vi "StellarNet_Raman_Obtain_Spectra_MODIFIED.vi"() -> ()   [LabVIEW 2014]
uses:
  Environmental Chamber LabVIEW and Instruments/Environment_Instrument_VIs/SpectraWiz_LabVIEW-1chan-free 2013.llb/StellarNet SpectraWiz Globals.vi
panel:
  in  "Channel to monitor":i8=1 min=1 max=1
  out "?":T1(graph)
  in  "Use Dark":bool
  in  "Take Dark":bool
  in  "Take Reference":bool
  in  "Mode Selection":u16(ring) items=["Scope Mode", "Absorbance Mode", "Transmission Mode", "Radiometer Mode"]
  in  "View Data File":bool
  in  "Open Data File":bool
  out "?":T1(graph)
  in  "Reset Coefficients":bool
  in  "Drift Correct":bool
  in  "View Snapshot":bool
  in  "Take Snapshot":bool
  in  "Channel":u8=1 min=1 max=1
  in  "Operating Parameters":T2(array[cluster]) {"Digitizer Clock Rate Setting" min=1 max=3; "Optical Smoothing Level" min=0 max=4 step=1; "Number of Scans to Average" min=1 max=10000 step=1}
  out "Number of Channels:":i32
  in  "Clear History":bool
  out "?":T1(graph)
  in  "Create and Log to Time Series Log File":bool
  out "ChartView":T3(graph)
  out "Time [s]":dbl format="%.2f"
  out "Data File":cluster{dbl[], dbl[]}
  out "Cursor Indices":i32[](array[numeric])
  in  "Stop Program":bool
  # "``"
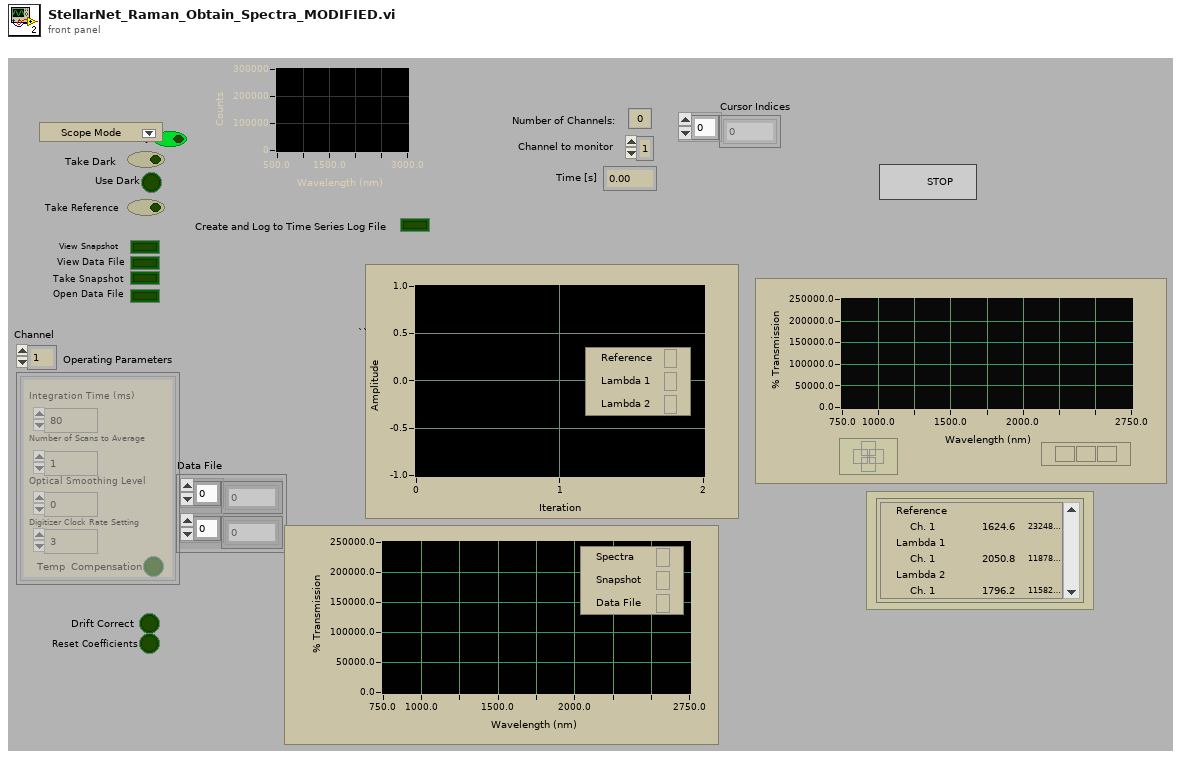
[diagram p1: front panel]
types:
  T1 = cluster{"Spectrometer Wavelengths":dbl[], dbl[]}[]
  T2 = cluster{"Integration Time (ms)":i32, "Number of Scans to Average":i32, "Optical Smoothing Level":i32, "Digitizer Clock Rate Setting":i32, "Temp  Compensation ":bool}[]
  T3 = cluster{"Cursor Y":dbl, "Cursor Y":dbl, "Cursor Y":dbl}
  T4 = cluster{"Cursor Y":dbl, "Cursor Y":dbl, "Cursor Y":dbl}[]
  T5 = cluster{"Coefficients":ext[], "Wavelengths":dbl[]}[]
  T6 = cluster{"[0]":dbl, "[1]":dbl, "[2]":dbl, "[3]":dbl, "[4]":dbl, "[5]":dbl, "[6]":dbl, "[7]":dbl, "[8]":dbl}
  T7 = cluster{"Minimum":dbl, "Maximum":dbl, "Increment":dbl, "Minor Incr":dbl, "Start":dbl}
  T8 = cluster{"Integration Time (ms)":i32, "Number of Scans to Average":i32, "Optical Smoothing Level":i32, "Digitizer Clock Rate Setting":i32, "Temp  Compensation ":bool}
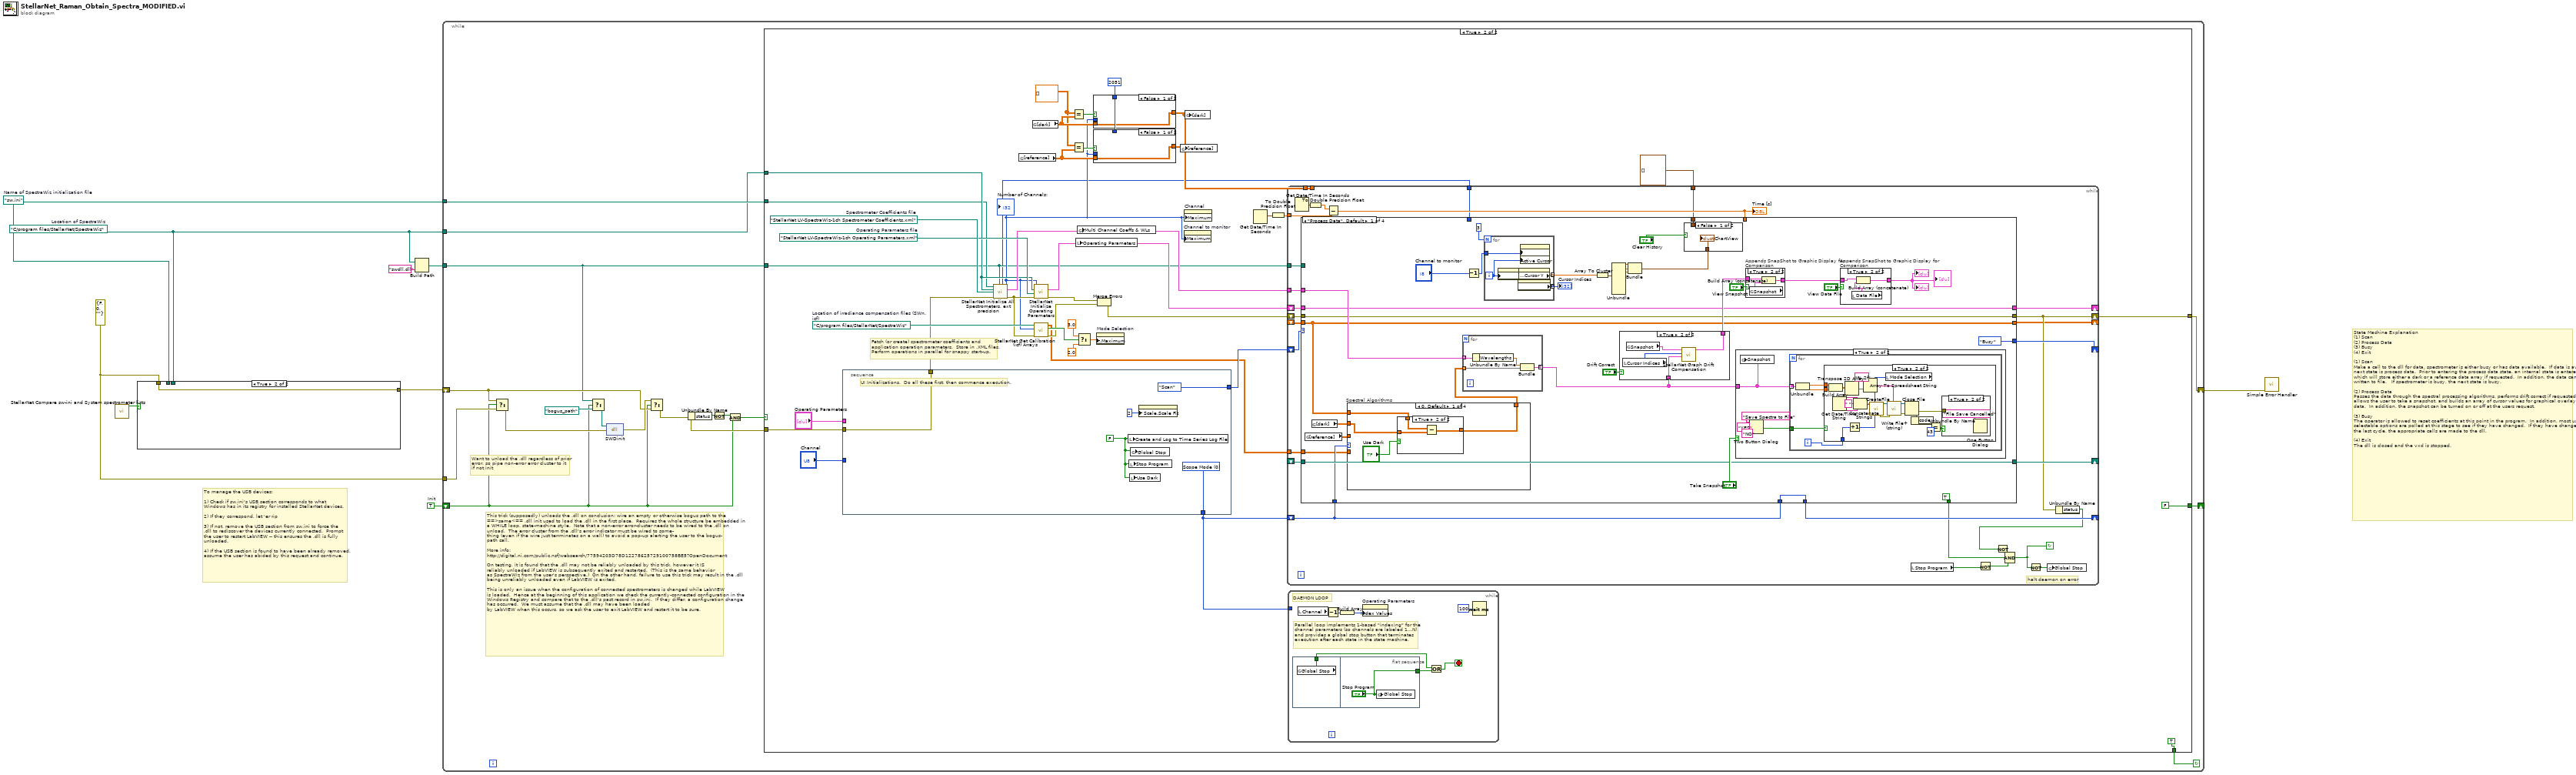
[diagram p0: block diagram]
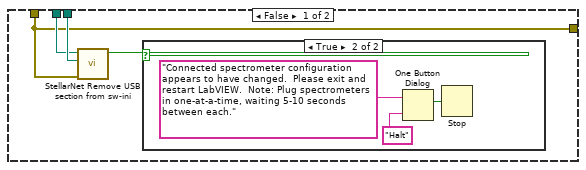
[diagram p2: hidden frame]
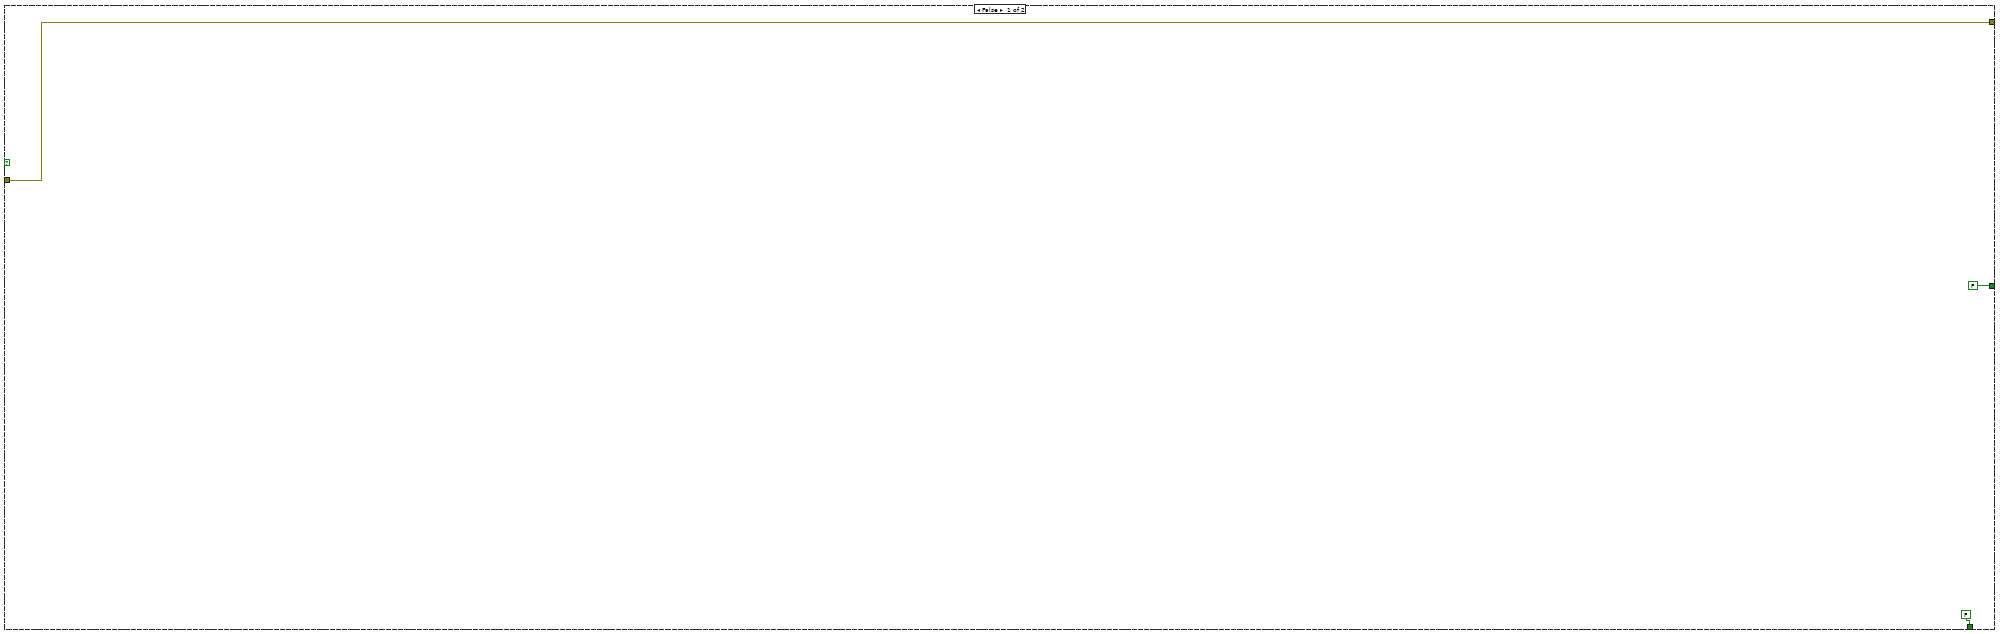
[diagram p4: hidden frame]
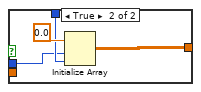
[diagram p5: hidden frame]
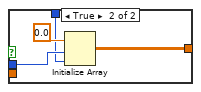
[diagram p6: hidden frame]
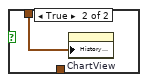
[diagram p7: hidden frame]
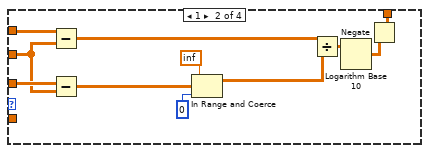
[diagram p12: hidden frame]
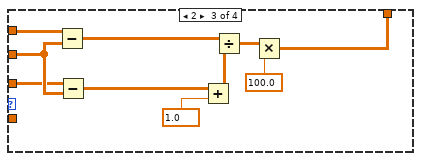
[diagram p13: hidden frame]
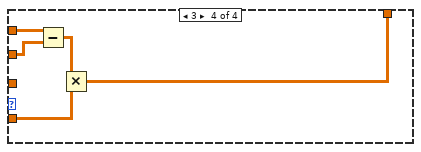
[diagram p14: hidden frame]
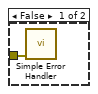
[diagram p17: hidden frame]
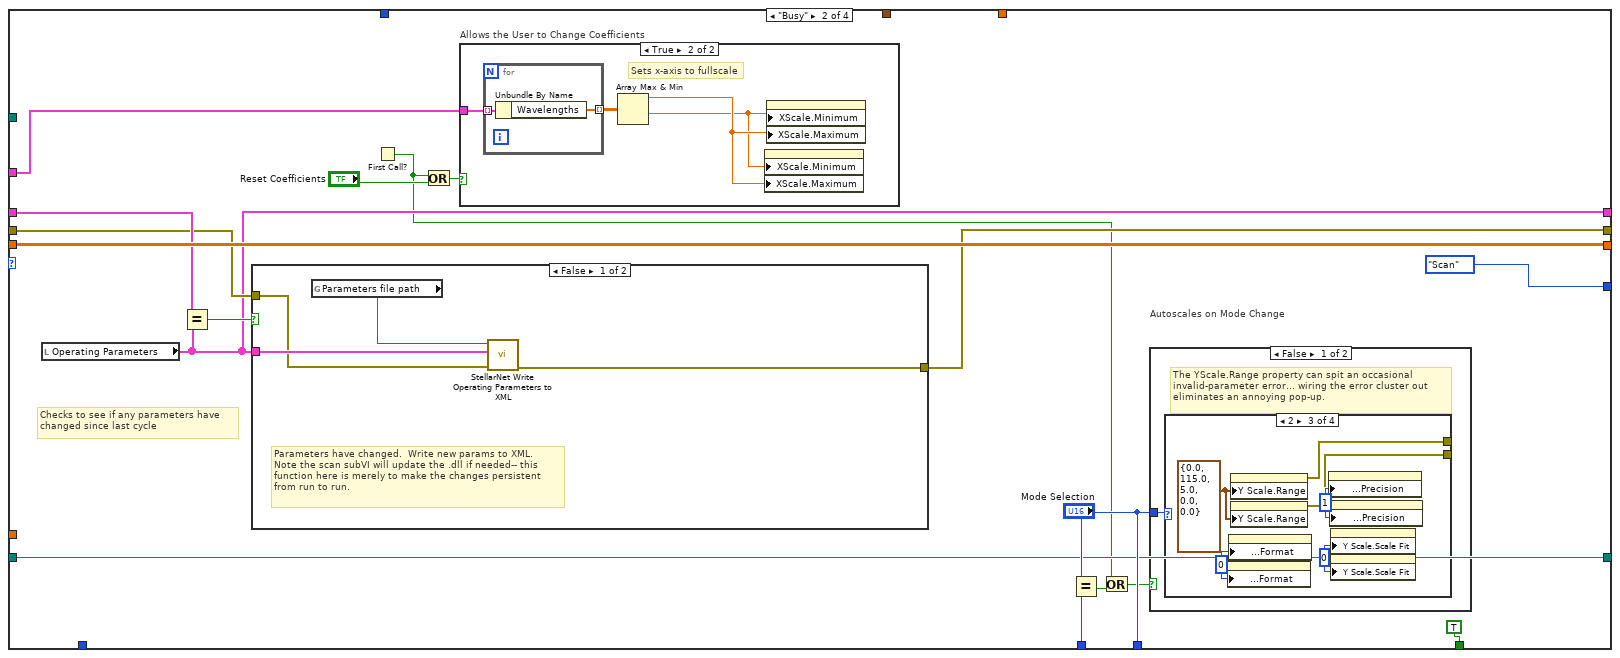
[diagram p18: hidden frame]
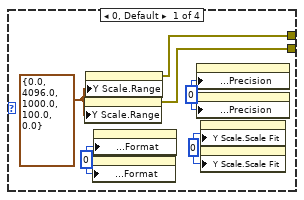
[diagram p20: hidden frame]
diagram:
  w4 = path "C:/program files/StellarNet/SpectraWiz"  # Location of SpectraWiz
  w8 = path "sw.ini"  # Name of SpectraWiz initialization file
  w6 = errorcluster {"status"=FALSE, "code"=0, "source"=""} ("error in (no error)")
  w9 = TRUE  # Init
  # "To manage the USB devices:\n\n1) Check if sw.ini's USB section corresponds to what\nWindows has in its registry for installed StellarNet devices.\n\n2) If they correspond, let 'er rip\n\n3) If not, remove the USB section from sw.ini to force the \n.dll to rediscover the devices currently connected.  Prompt\nthe user to restart LabVIEW -- this ensures the .dll is fully\nunloaded.  \n\n4) If the USB section is found to have been already removed, \nassume the user has abided by this request and continue."
  # "State Machine Explanation\n(1) Scan\n(2) Process Data\n(3) Busy\n(4) Exit\n\n(1) Scan\nMake a call to the dll for data, spectrometer is either busy or has data available.  If data is available, next state is process data.  Prior to entering the process data state, an internal state is entered which will store either a dark or a reference data array if requested.  In addition, the data can be written to file.   If spectrometer is busy, the next state is busy.\n\n(2) Process Data\nPasses the data through the spectral processing algorithms, performs drift correct if requested, allows the user to take a snapshot, and builds an array of cursor values for graphical overlay on the data.  In addition, the snapshot can be turned on or off at the users request.\n\n(3) Busy\nThe operator is allowed to reset coefficients at this point in the program.  In addition, most user selectable options are polled at this stage to see if they have changed.  If they have changed since the last cycle, the appropriate calls are made to the dll.\n\n(4) Exit\nThe dll is closed and the vxd is stopped."
  n1 = call "StellarNet Compare sw-ini and System spectrometer lists.vi"() -> ("Configs\nAgree"=w5:bool)  [unwired: 11 in]
  n2 = case shown="True" w5 {
    tunnel: w6 -> [w11 w17]
    tunnel: w4 -> [w13 _]
    tunnel: w8 -> [w12 _]
    tunnel: [w11 w17] -> w7
    frame False {
      n3 = call "StellarNet Remove USB section from sw-ini.vi"("error in (no error)"=w11, "Location of SpectraWiz"=w13, "Name of SpectraWiz initialization file"=w12) -> ("USB section found?"=w10:bool)  [unwired: 7 in, 1 out]
      n4 = case shown="True" w10 {
        frame False {
        }
        frame True {
          n5 = One Button Dialog(message="Connected spectrometer configuration appears to have changed.  Please exit and restart LabVIEW.  Note: Plug spectrometers in one-at-a-time, waiting 5-10 seconds between each.", button name ("OK")="Halt") -> (true=w15:bool)
          n6 = Stop(stop? (T)=w15) -> ()
        }
      }
    }
    frame True {
    }
  }
  n7 = Build Path(base path=w4, name or relative path="swdll.dll") -> (appended path=w2:path)
  n8 = while {
    shift-right: [w34] -> _
    shift-left: w9 -> [w20]
    tunnel: w8 -> [w27]
    tunnel: w4 -> [w19]
    shift-right: [w26] -> w1
    shift-left: w7 -> [w21]
    tunnel: w6 -> [w25]
    tunnel: w2 -> [w18]
    stop <- w33 continue-if-true
    # "This trick (supposedly) unloads the .dll on conclusion: wire an empty or otherwise bogus path to the ==>same<== .dll init used to load the .dll in the first place.  Requires the whole structure be embedded in a WHILE loop, state-machine style.  Note that a non-error error-cluster needs to be wired to the .dll on unload.  The error cluster from the .dll's error indicator must be wired to some-\nthing (even if the wire just terrminates on a wall) to avoid a pop-up alerting the user to the bogus-\npath call.\n\nMore info:\nhttp://digital.ni.com/public.nsf/websearch/77594203D78D12278625729100758BE5?OpenDocument\n\nOn testing, it is found that the .dll may not be reliably unloaded by this trick, however it IS\nreliably unloaded if LabVIEW is subsequently exited and restarted.  (This is the same behavior\nas SpectraWiz from the user's perspective.)  On the other hand, failure to use this trick may result in the .dll being unreliably unloaded even if LabVIEW is exited.\n\nThis is only an issue when the configuration of connected spectrometers is changed while LabVIEW\nis loaded.  Hence at the beginning of this application we check the currently-connected configuration in the Windows Registry and compare that to the .dll's past record in sw.ini.  If they differ, a configuration change has occurred.  We must assume that the .dll may have been loaded \nby LabVIEW when this occurs, so we ask the user to exit LabVIEW and restart it to be sure."
    # "Want to unload the .dll regardless of prior\nerror, so pipe non-error error cluster to it\nif not init"
    n9 = Select(t=w21, s=w20, f=w25) -> (s? t:f=w24:errorcluster)
    n10 = Select(t=w18, s=w20, f=path "bogus_path" ("reference")) -> (s? t:f=w31:path)
    n11 = dll-call lib="C:/Program Files/StellarNet/SpectraWiz/swdll.dll" fn="SWDinit" label="init"(path in=w31, error in=w24) -> (error out=w23:errorcluster)  [unwired: 2 in, 1 out]
    n12 = Select(t=w23, s=w20, f=w21) -> (s? t:f=w22:errorcluster)
    n13 = Unbundle By Name(w22) -> ("status"=w29:bool)
    n14 = Not(x=w29) -> (.not. x?=w30:bool)
    n15 = And(x=w30, y=w20) -> (x .and. y?=w28:bool)
    n16 = case shown="True" w28 {
      tunnel: [w35 w42] -> w26
      tunnel: w22 -> [w35 w48]
      tunnel: [FALSE ("Init") FALSE ("Init")] -> w34
      tunnel: [FALSE TRUE] -> w33
      tunnel: w19 -> [_ w44]
      tunnel: w27 -> [_ w43]
      tunnel: w18 -> [_ w39]
      frame False {
      }
      frame True {
        w49 = 2051 ("dimension size")
        w54 = sgl[][] [] ("[dark]")
        w72 = path "C:/program files/StellarNet/SpectraWiz"  # Location of irradiance compensation files (SWn.icf)
        w73 = path "StellarNet LV-SpectraWiz-1ch Operating Parameters.xml"  # Operating Parameters file
        w74 = path "StellarNet LV-SpectraWiz-1ch Spectrometer Coefficients.xml"  # Spectrometer Coefficients file
        # "Fetch (or create) spectrometer coefficients and\napplication operation parameters.  Store in .XML files.\nPerform operations in parallel for snappy start-up."
        n17 = stacked-sequence {
          tunnel: [w99] -> w57
          tunnel: [enum16{"Process Data", "Busy", "Exit", "Scan"}."Scan" ("Enum")] -> w64
          tunnel: [w97] -> w45
          tunnel: "Channel" -> [_]
          tunnel: "Operating Parameters" -> [_]
          tunnel: w48 -> [w97]
          frame #0 {
            w99 = u16 0 items=["Scope Mode", "Absorbance Mode", "Transmission Mode", "Radiometer Mode"] ("Mode Selection")
            w96 = FALSE ("File Stamp")
            # "UI Initializations.  Do all these first, then commence execution."
            n18 = local write "Create and Log to Time Series Log File"(w96) -> ()
            n19 = local write "Stop Program"(w96) -> ()
            n20 = local write "Use Dark"(w96) -> ()
            n21 = global write "StellarNet SpectraWiz Globals.vi" "Global Stop"(w96) -> ()
            n22 = property class="XYGraph (strict)"("Y Scale.Scale Fit"=u8 2) -> ()  [unwired: 2 in, 2 out]
          }
        }
        n23 = call "StellarNet Initialize All Spectrometers, ext precision.vi"("Path of swdll.dll"=w39, "error in"=w45, "Spectrometer Coefficients file"=w74, "Location of SpectraWiz"=w44, "Name of SpectraWiz initialization file"=w43) -> ("error out"=w71:errorcluster, "Multi Channel Coeffs & WLs"=w58:T5, "Number of Channels"=w40:i32, "Detector Types"=w38:u16[])  [unwired: 2 in, 1 out]
        "Number of Channels:" <- w40
        n24 = global read "StellarNet SpectraWiz Globals.vi" "[reference]"() -> (w52:sgl[][])
        n25 = global read "StellarNet SpectraWiz Globals.vi" "[dark]"() -> (w55:sgl[][])
        n26 = call "StellarNet Initialize Operating Parameters.vi"("error in"=w71, "Spectrometer Coefficients file"=w73, "Location of SpectraWiz"=w44, "Number of Channels"=w40) -> ("error out"=w66:errorcluster, "Operating Parameters"=w61:T2)  [unwired: 6 in]
        n27 = call "StellarNet Get Calibration (icf) Arrays.vi"("error in (no error)"=w71, "Number of Channels"=w40, "directory path"=w72) -> ("error out"=w65:errorcluster, ".icf found for\nat least one channel"=w67:bool, "N x Compensation Array"=w62:dbl[][])  [unwired: 6 in]
        n28 = Equal?(x=w54, y=w55) -> (x = y?=w56:bool)
        n29 = Equal?(x=w54, y=w52) -> (x = y?=w53:bool)
        n30 = local write "Operating Parameters"(w61) -> ()
        n31 = global write "StellarNet SpectraWiz Globals.vi" "Multi Channel Coeffs & WLs"(w58) -> ()
        n32 = Select(t=3.0 ("Data Range:Maximum"), s=w67, f=2.0 ("Data Range:Maximum")) -> (s? t:f=w70:dbl)
        n33 = case shown="False" w56 {
          tunnel: [w82 w86] -> w51
          tunnel: w55 -> [w82 _]
          tunnel: w40 -> [_ w84]
          tunnel: w49 -> [_ w83]
          frame False {
          }
          frame True {
            n34 = Initialize Array(0.0, w84, w83) -> (w86:dbl[][])
          }
        }
        n35 = case shown="False" w53 {
          tunnel: [w77 w81] -> w50
          tunnel: w52 -> [w77 _]
          tunnel: w40 -> [_ w78]
          tunnel: w49 -> [_ w79]
          frame False {
          }
          frame True {
            n36 = Initialize Array(0.0, w78, w79) -> (w81:dbl[][])
          }
        }
        n37 = property on="Mode Selection" class="Ring (strict)"("Data Range:Maximum"=w70) -> ()  [unwired: 2 in, 2 out]
        n38 = Merge Errors(w66, w65) -> (w63:errorcluster)
        n39 = global write "StellarNet SpectraWiz Globals.vi" "[reference]"(w50) -> ()
        n40 = property on="Channel to monitor" class="DigNum (strict)"("Maximum"=w40) -> ()  [unwired: 2 in, 2 out]
        n41 = property on="Channel" class="DigNum (strict)"("Maximum"=w40) -> ()  [unwired: 2 in, 2 out]
        n42 = global write "StellarNet SpectraWiz Globals.vi" "[dark]"(w51) -> ()
        n43 = Get Date/Time In Seconds() -> (seconds since 1Jan1904=w75:timestamp)
        n44 = To Double Precision Float(number=w75) -> (double precision float=w76:dbl)
        n45 = while {
          tunnel: w76 -> [w127]
          shift-right: [w126] -> _
          shift-left: w57 -> [w119]
          shift-right: [w124] -> _
          shift-left: w64 -> [w125]
          shift-right: [w121] -> _
          shift-left: _ -> [w122]
          shift-right: [w117] -> w42
          shift-left: w63 -> [w118]
          shift-right: [w116] -> _
          shift-left: _ -> [w115]
          tunnel: w58 -> [w114]
          tunnel: w62 -> [w113]
          tunnel: w51 -> [_]
          tunnel: w50 -> [_]
          shift-right: [w104] -> _
          shift-left: w61 -> [w112]
          tunnel: T4 [] ("History Data") -> [w103]
          tunnel: w39 -> [w102]
          tunnel: w38 -> [w101]
          stop <- w108 continue-if-true
          # "halt daemon on error"
          n46 = Get Date/Time In Seconds() -> (seconds since 1Jan1904=w120:timestamp)
          n47 = To Double Precision Float(number=w120) -> (double precision float=w128:dbl)
          n48 = Subtract(x=w128, y=w127) -> (x-y=w123:dbl)
          "Time [s]" <- w123
          n49 = case shown="\"Process Data\", Default" w125 {
            tunnel: w119 -> [w154 w269 w313 w335]
            tunnel: [w154 "Mode Selection" w313 w335] -> w126
            tunnel: [enum16{"Process Data", "Busy", "Exit", "Scan"}."Busy" ("Enum") enum16{"Process Data", "Busy", "Exit", "Scan"}."Scan" ("Enum") enum16{"Process Data", "Busy", "Exit", "Scan"}."Process Data" ("Enum") enum16{"Process Data", "Busy", "Exit", "Scan"}."Process Data" ("Enum")] -> w124
            tunnel: [TRUE TRUE FALSE TRUE] -> w109
            tunnel: [w142 w263 w308 w322] -> w116
            tunnel: w123 -> [_ _ _ w343]
            tunnel: w122 -> [w149 w265 w311 w344]
            tunnel: [w149 w265 w311 w342] -> w121
            tunnel: w119 -> [w148 _ _ _]
            tunnel: w112 -> [w136 w262 w306 w327]
            tunnel: w118 -> [w137 w260 w307 w324]
            tunnel: [w137 w259 w307 w329] -> w117
            tunnel: w115 -> [w142 w263 w308 _]
            tunnel: w114 -> [w143 w264 _ _]
            tunnel: w113 -> [w140 _ _ _]
            tunnel: [w136 w258 w306 w327] -> w104
            tunnel: w103 -> [w134 _ _ _]
            tunnel: w102 -> [_ _ _ w323]
            tunnel: w101 -> [_ _ _ w318]
            frame "Process Data", Default {
              n50 = global read "StellarNet SpectraWiz Globals.vi" "[reference]"() -> (w144:sgl[][])
              n51 = global read "StellarNet SpectraWiz Globals.vi" "[dark]"() -> (w145:sgl[][])
              n52 = case "Spectral Algorithms" shown="0, Default" w148 {
                tunnel: [w189 w203 w211 w217] -> w141
                tunnel: w142 -> [w188 w202 w208 w219]
                tunnel: w145 -> [w187 w198 w206 w216]
                tunnel: w144 -> [_ w199 w205 _]
                tunnel: w140 -> [_ _ _ w215]
                frame 0, Default {
                  n53 = case shown="True" "Use Dark" {
                    tunnel: [w190 w193] -> w189
                    tunnel: w188 -> [w190 w192]
                    tunnel: w187 -> [_ w191]
                    frame False {
                    }
                    frame True {
                      n54 = Subtract(x=w192, y=w191) -> (x-y=w193:sgl[][])
                    }
                  }
                }
                frame 1 {
                  n55 = Subtract(x=w202, y=w198) -> (x-y=w201:sgl[][])
                  n56 = Subtract(x=w199, y=w198) -> (x-y=w195:sgl[][])
                  n57 = In Range and Coerce(upper limit=inf, x=w195, lower limit=0) -> (coerced(x)=w194:dbl[][])  [unwired: 1 out]
                  n58 = Divide(x=w201, y=w194) -> (x/y=w200:dbl[][])
                  n59 = Logarithm Base 10(1:w200) -> (0:w204:dbl[][])
                  n60 = Negate(x=w204) -> (-x=w203:dbl[][])
                }
                frame 2 {
                  n61 = Subtract(x=w208, y=w206) -> (x-y=w214:sgl[][])
                  n62 = Subtract(x=w205, y=w206) -> (x-y=w209:sgl[][])
                  n63 = Add(x=w209, y=sgl 1.0) -> (x+y=w207:sgl[][])
                  n64 = Divide(x=w214, y=w207) -> (x/y=w213:sgl[][])
                  n65 = Multiply(x=w213, y=sgl 100.0) -> (x*y=w211:sgl[][])
                }
                frame 3 {
                  n66 = Subtract(x=w219, y=w216) -> (x-y=w218:sgl[][])
                  n67 = Multiply(x=w218, y=w215) -> (x*y=w217:dbl[][])
                }
              }
              n68 = for {
                tunnel: w143 -> [w172] mode=indexing
                tunnel: w141 -> [w170] mode=indexing
                tunnel: [w169] -> w139 mode=indexing
                n69 = Unbundle By Name(w172) -> ("Wavelengths"=w171:dbl[])
                n70 = Bundle("Wavelengths"=w171, w170) -> (w169:cluster{"Wavelengths":dbl[], dbl[]})  [unwired: 1 in]
              }
              n71 = Decrement(x="Channel to monitor") -> (x-1=w129:i8)
              n72 = for {
                N: 3 -> [_]
                tunnel: [w166] -> w159 mode=indexing
                tunnel: [w164] -> w131 mode=indexing
                tunnel: w129 -> [w162]
                i -> [w163]
                n73 = property class="XYGraph (strict)"("Active Cursor"=w163) -> (error out=w165:errorcluster)  [unwired: 2 in, 1 out]
                n74 = property class="XYGraph (strict)"(error in=w165) -> ("Cursor.Cursor Index"=w164:i32)  [unwired: 1 in, 2 out]
                n75 = property class="XYGraph (strict)"(error in=w165) -> ("Cursor.Cursor Position:Cursor Y"=w166:dbl)  [unwired: 1 in, 2 out]
                n76 = property class="XYGraph (strict)"("Cursor.Cursor Plot"=w162, "Active Cursor"=w163) -> ()  [unwired: 2 in, 2 out]
              }
              "Cursor Indices" <- w131
              n77 = Array To Cluster(array=w159) -> (cluster=w158:T6)
              n78 = Unbundle(w158) -> ("[0]"=w157:dbl, "[1]"=w156:dbl, "[2]"=w155:dbl)  [unwired: 6 out]
              n79 = case shown="True" "Drift Correct" {
                tunnel: w139 -> [w177 w181]
                tunnel: [w177 w178] -> w151
                frame False {
                }
                frame True {
                  n80 = local read "Cursor Indices"() -> (w179:i32[])
                  n81 = global read "StellarNet SpectraWiz Globals.vi" "Snapshot"() -> (w180:cluster{"Wavelengths":dbl[], sgl[]}[])
                  n82 = call "StellarNet Graph Drift Compensation.vi"("Current Graph"=w181, "Cursor Indices"=w179, "Snapshot"=w180) -> ("De-Drifted Current Graph"=w178:cluster{"Wavelengths":dbl[], sgl[]}[])  [unwired: 8 in]
                }
              }
              n83 = Bundle("[0]"=w157, "[1]"=w156, "[2]"=w155) -> (w133:cluster{"[0]":dbl, "[1]":dbl, "[2]":dbl})  [unwired: 1 in]
              n84 = case shown="False" "Clear History" {
                tunnel: w134 -> [_ w168]
                tunnel: w133 -> [w167 _]
                frame False {
                  "ChartView" <- w167
                }
                frame True {
                  n85 = property on="ChartView" class="WFChart (strict)"("History Data"=w168) -> ()  [unwired: 2 in, 2 out]
                }
              }
              n86 = case shown="True" "Take Snapshot" {
                tunnel: w139 -> [_ w220]
                frame False {
                }
                frame True {
                  n87 = global write "StellarNet SpectraWiz Globals.vi" "Snapshot"(w220) -> ()
                  n88 = Two Button Dialog(message="Save Spectra to File", 1:"NO" ("F button name (\"Cancel\")"), 2:"YES" ("T button name (\"OK\")")) -> (T button?=w224:bool)
                  n89 = for {
                    tunnel: w224 -> [w229]
                    tunnel: w220 -> [w228] mode=indexing
                    i -> [w225]
                    n90 = Unbundle(w228) -> ("Wavelengths"=w227:dbl[], w226:dbl[])
                    n91 = case shown="True" w229 {
                      tunnel: w227 -> [_ w240]
                      tunnel: w226 -> [_ w239]
                      tunnel: w225 -> [_ w231]
                      frame False {
                      }
                      frame True {
                        n92 = Build Array(w240, w239) -> (w233:dbl[][])
                        n93 = Get Date/Time String() -> (date string=w246:string, time string=w245:string)  [unwired: 3 in]
                        n94 = Transpose 2D Array(2D array=w233) -> (transposed array=w241:dbl[][])
                        n95 = Increment(x=w231) -> (x+1=w230:i32)
                        n96 = Concatenate Strings(w246, " ", w245) -> (w247:string)
                        n97 = Array To Spreadsheet String(array=w241, 3:"%.2f" ("format string")) -> (spreadsheet string=w242:string)  [unwired: 1 in]
                        n98 = local read "Mode Selection"() -> (w232:u16)
                        n99 = call "CreateFile.vi"("Time Stamp"=w247, "Mode Selection"=w232, "Channel (1-based)"=w230) -> ("Refnumber"=w249:refnum<file>, "Error Out"=w248:errorcluster)  [unwired: 2 in, 2 out]
                        n100 = call <vilib>:"Write File+ (string).vi"("string"=w242, "error in (no error)"=w248, "refnum"=w249) -> ("error out"=w238:errorcluster, "dup refnum"=w250:refnum<file>)  [unwired: 4 in, 1 out]
                        n101 = Close File(refnum=w250, error in=w238) -> (error out=w234:errorcluster)  [unwired: 1 out]
                        n102 = Unbundle By Name(w234) -> ("code"=w236:i32)
                        n103 = Equal?(x=w236, y=43) -> (x = y?=w235:bool)
                        n104 = case shown="True" w235 {
                          tunnel: w234 -> [w251 _]
                          frame False {
                            n105 = call <vilib>:"Simple Error Handler.vi"("error in (no error)"=w251) -> ()  [unwired: 4 in, 5 out]
                          }
                          frame True {
                            n106 = One Button Dialog(message="File Save Cancelled") -> ()  [unwired: 1 in, 1 out]
                          }
                        }
                      }
                    }
                  }
                }
              }
              n107 = case "Appends SnapShot to Graphic Display for Comparison" shown="True" "View Snapshot" {
                tunnel: w151 -> [w182 w185]
                tunnel: [w182 w183] -> w138
                frame False {
                }
                frame True {
                  n108 = global read "StellarNet SpectraWiz Globals.vi" "Snapshot"() -> (w184:cluster{"Wavelengths":dbl[], sgl[]}[])
                  n109 = Build Array (concatenate)(w185, w184) -> (w183:cluster{"Wavelengths":dbl[], dbl[]}[])
                }
              }
              n110 = case "Appends SnapShot to Graphic Display for Comparison" shown="True" "View Data File" {
                tunnel: w138 -> [w173 w176]
                tunnel: [w173 w174] -> w146
                frame False {
                }
                frame True {
                  n111 = local read "Data File"() -> (w175:cluster{dbl[], dbl[]})
                  n112 = Build Array (concatenate)(w176, w175) -> (w174:cluster{"Wavelengths":dbl[], dbl[]}[])
                }
              }
              "?" <- w146
              "?" <- w146
              "?" <- w146
            }
            frame "Busy" {
              # "Checks to see if any parameters have \nchanged since last cycle"
              n113 = local read "Operating Parameters"() -> (w258:T2)
              n114 = Equal?(x=w262, y=w258) -> (x = y?=w261:bool)
              n115 = case shown="False" w261 {
                tunnel: w258 -> [w272 _]
                tunnel: w260 -> [w271 w274]
                tunnel: [w270 w274] -> w259
                frame False {
                  # "Parameters have changed.  Write new params to XML.\nNote the scan subVI will update the .dll if needed-- this\nfunction here is merely to make the changes persistent\nfrom run to run."
                  n116 = global read "StellarNet SpectraWiz Globals.vi" "Parameters file path"() -> (w273:path)
                  n117 = call "StellarNet Write Operating Parameters to XML.vi"("error in (no error)"=w271, "Operating Parameters"=w272, "XML File Path"=w273) -> ("error out"=w270:errorcluster)  [unwired: 8 in]
                }
                frame True {
                  # "Parameters are the same.  Do nothing."
                }
              }
              n118 = First Call?() -> (First Call?: T/F=w254:bool)
              n119 = Or(x=w254, y="Reset Coefficients") -> (x .or. y?=w256:bool)
              n120 = case "Allows the User to Change Coefficients" shown="True" w256 {
                tunnel: w264 -> [_ w303]
                frame False {
                }
                frame True {
                  # "Sets x-axis to fullscale"
                  n121 = for {
                    tunnel: w303 -> [w305] mode=indexing
                    tunnel: [w304] -> w302 mode=indexing
                    n122 = Unbundle By Name(w305) -> ("Wavelengths"=w304:dbl[])
                  }
                  n123 = Array Max & Min(array=w302) -> (max value=w301:dbl, min value=w300:dbl)  [unwired: 2 out]
                  n124 = property class="XYGraph (strict)"("XScale.Minimum"=w300, "XScale.Maximum"=w301) -> ()  [unwired: 2 in, 2 out]
                  n125 = property class="XYGraph (strict)"("XScale.Minimum"=w300, "XScale.Maximum"=w301) -> ()  [unwired: 2 in, 2 out]
                }
              }
              n126 = Equal?(x="Mode Selection", y=w269) -> (x = y?=w255:bool)
              n127 = Or(x=w254, y=w255) -> (x .or. y?=w253:bool)
              n128 = case "Autoscales on Mode Change" shown="False" w253 {
                tunnel: "Mode Selection" -> [w275 _]
                frame False {
                  # "The YScale.Range property can spit an occasional \ninvalid-parameter error... wiring the error cluster out \neliminates an annoying pop-up."
                  n129 = case shown="2" w275 {
                    tunnel: [w277 w283 w289 w295] -> _
                    tunnel: [w276 w282 w288 w294] -> _
                    frame 0, Default {
                      w278 = 0
                      w279 = T7 {"Minimum"=0.0, "Maximum"=4096.0, "Increment"=1000.0, "Minor Incr"=100.0, "Start"=0.0} ("Y Scale.Range")
                      w281 = 0
                      w280 = u8 0 ("Y Scale.Scale Fit")
                      n130 = property class="XYGraph (strict)"("Y Scale.Range"=w279) -> (error out=w276:errorcluster)  [unwired: 2 in, 1 out]
                      n131 = property class="XYGraph (strict)"("Y Scale.Range"=w279) -> (error out=w277:errorcluster)  [unwired: 2 in, 1 out]
                      n132 = property class="XYGraph (strict)"("Y Scale.Format & Precision:Format"=w278) -> ()  [unwired: 2 in, 2 out]
                      n133 = property class="XYGraph (strict)"("Y Scale.Format & Precision:Format"=w278) -> ()  [unwired: 2 in, 2 out]
                      n134 = property class="XYGraph (strict)"("Y Scale.Format & Precision:Precision"=w281) -> ()  [unwired: 2 in, 2 out]
                      n135 = property class="XYGraph (strict)"("Y Scale.Format & Precision:Precision"=w281) -> ()  [unwired: 2 in, 2 out]
                      n136 = property class="XYGraph (strict)"("Y Scale.Scale Fit"=w280) -> ()  [unwired: 2 in, 2 out]
                      n137 = property class="XYGraph (strict)"("Y Scale.Scale Fit"=w280) -> ()  [unwired: 2 in, 2 out]
                    }
                    frame 1 {
                      w284 = 0
                      w287 = 1
                      w286 = T7 {"Minimum"=0.0, "Maximum"=3.0, "Increment"=0.001, "Minor Incr"=0.0, "Start"=0.0} ("Y Scale.Range")
                      w285 = u8 0 ("Y Scale.Scale Fit")
                      n138 = property class="XYGraph (strict)"("Y Scale.Range"=w286) -> (error out=w282:errorcluster)  [unwired: 2 in, 1 out]
                      n139 = property class="XYGraph (strict)"("Y Scale.Range"=w286) -> (error out=w283:errorcluster)  [unwired: 2 in, 1 out]
                      n140 = property class="XYGraph (strict)"("Y Scale.Format & Precision:Format"=w284) -> ()  [unwired: 2 in, 2 out]
                      n141 = property class="XYGraph (strict)"("Y Scale.Format & Precision:Format"=w284) -> ()  [unwired: 2 in, 2 out]
                      n142 = property class="XYGraph (strict)"("Y Scale.Format & Precision:Precision"=w287) -> ()  [unwired: 2 in, 2 out]
                      n143 = property class="XYGraph (strict)"("Y Scale.Format & Precision:Precision"=w287) -> ()  [unwired: 2 in, 2 out]
                      n144 = property class="XYGraph (strict)"("Y Scale.Scale Fit"=w285) -> ()  [unwired: 2 in, 2 out]
                      n145 = property class="XYGraph (strict)"("Y Scale.Scale Fit"=w285) -> ()  [unwired: 2 in, 2 out]
                    }
                    frame 2 {
                      w290 = T7 {"Minimum"=0.0, "Maximum"=115.0, "Increment"=5.0, "Minor Incr"=0.0, "Start"=0.0} ("Y Scale.Range")
                      w291 = 0
                      w293 = 1
                      w292 = u8 0 ("Y Scale.Scale Fit")
                      n146 = property class="XYGraph (strict)"("Y Scale.Format & Precision:Format"=w291) -> ()  [unwired: 2 in, 2 out]
                      n147 = property class="XYGraph (strict)"("Y Scale.Format & Precision:Format"=w291) -> ()  [unwired: 2 in, 2 out]
                      n148 = property class="XYGraph (strict)"("Y Scale.Range"=w290) -> (error out=w289:errorcluster)  [unwired: 2 in, 1 out]
                      n149 = property class="XYGraph (strict)"("Y Scale.Range"=w290) -> (error out=w288:errorcluster)  [unwired: 2 in, 1 out]
                      n150 = property class="XYGraph (strict)"("Y Scale.Format & Precision:Precision"=w293) -> ()  [unwired: 2 in, 2 out]
                      n151 = property class="XYGraph (strict)"("Y Scale.Format & Precision:Precision"=w293) -> ()  [unwired: 2 in, 2 out]
                      n152 = property class="XYGraph (strict)"("Y Scale.Scale Fit"=w292) -> ()  [unwired: 2 in, 2 out]
                      n153 = property class="XYGraph (strict)"("Y Scale.Scale Fit"=w292) -> ()  [unwired: 2 in, 2 out]
                    }
                    frame 3 {
                      w296 = 1
                      w297 = T7 {"Minimum"=0.0, "Maximum"=1.0, "Increment"=0.1, "Minor Incr"=0.01, "Start"=0.0} ("Y Scale.Range")
                      w299 = 2
                      w298 = u8 0 ("Y Scale.Scale Fit")
                      n154 = property class="XYGraph (strict)"("Y Scale.Range"=w297) -> (error out=w294:errorcluster)  [unwired: 2 in, 1 out]
                      n155 = property class="XYGraph (strict)"("Y Scale.Range"=w297) -> (error out=w295:errorcluster)  [unwired: 2 in, 1 out]
                      n156 = property class="XYGraph (strict)"("Y Scale.Format & Precision:Format"=w296) -> ()  [unwired: 2 in, 2 out]
                      n157 = property class="XYGraph (strict)"("Y Scale.Format & Precision:Format"=w296) -> ()  [unwired: 2 in, 2 out]
                      n158 = property class="XYGraph (strict)"("Y Scale.Format & Precision:Precision"=w299) -> ()  [unwired: 2 in, 2 out]
                      n159 = property class="XYGraph (strict)"("Y Scale.Format & Precision:Precision"=w299) -> ()  [unwired: 2 in, 2 out]
                      n160 = property class="XYGraph (strict)"("Y Scale.Scale Fit"=w298) -> ()  [unwired: 2 in, 2 out]
                      n161 = property class="XYGraph (strict)"("Y Scale.Scale Fit"=w298) -> ()  [unwired: 2 in, 2 out]
                    }
                  }
                }
                frame True {
                }
              }
            }
            frame "Exit" {
              n162 = local write "Create and Log to Time Series Log File"(FALSE ("File Stamp")) -> ()
            }
            frame "Scan" {
              # "Truncate return array for \nnumber of pixels in spectrum"
              n163 = case shown="True" "Open Data File" {
                frame False {
                }
                frame True {
                  n164 = call <vilib>:"Read Characters From File.vi"() -> ("character string"=w362:string)  [unwired: 6 in, 3 out]
                  n165 = Search and Replace String(replace all?=TRUE ("replace all? (F)"), input string=w362, search string="\r\n ", replace string="\r\n") -> (result string=w366:string)  [unwired: 4 in, 3 out]
                  n166 = Search and Replace String(replace all?=TRUE ("replace all? (F)"), input string=w366, search string="  ", replace string="\t") -> (result string=w370:string)  [unwired: 4 in, 3 out]
                  n167 = Spreadsheet String To Array(delimiter (Tab)="\t", format string="%f", spreadsheet string=w370) -> (array=w373:dbl[][])  [unwired: 1 in]
                  n168 = Transpose 2D Array(2D array=w373) -> (transposed array=w361:dbl[][])
                  n169 = Delete From Array(array=w361, index (col)=0 ("disabled index (col)")) -> (array with subset deleted=w358:dbl[][])  [unwired: 2 in, 1 out]
                  n170 = Delete From Array(array=w358, index (col)=0 ("disabled index (col)")) -> (array with subset deleted=w356:dbl[][])  [unwired: 2 in, 1 out]
                  n171 = Index Array(array=w356, index (row)=0) -> (element=w355:dbl[])  [unwired: 1 in]
                  n172 = Index Array(array=w356, index (row)=1) -> (element=w353:dbl[])  [unwired: 1 in]
                  n173 = Bundle(w355, w353) -> (→"Data File":cluster{dbl[], dbl[]})  [unwired: 1 in]
                }
              }
              n174 = local read "Channel"() -> (w319:u8)
              n175 = Decrement(x=w319) -> (x-1=w321:u8)
              n176 = Index Array(array=w327, index=w321) -> (element=w325:T8)
              n177 = Index Array(array=w318, index=w319) -> (element=w317:u16)
              n178 = case shown="5" w317 {
                tunnel: [2048 512 1024] -> w320
                frame 1, Default {
                }
                frame 5 {
                }
                frame 6 {
                }
              }
              n179 = Decrement(x=w320) -> (x-1=w316:i32)
              n180 = call "StellarNet Single-Channel Scan rev A.vi"("Path of sw.dll"=w323, "error in (no error)"=w324, "Operation Settings"=w325, "Channel (1-based)"=w319) -> ("error out"=w326:errorcluster, "buffer out"=w315:sgl[])  [unwired: 4 in, 2 out]
              n181 = Split 1D Array(array=w315, index=w316) -> (first subarray=w314:sgl[])  [unwired: 1 out]
              n182 = Build Array(w314) -> (w322:sgl[][])
              n183 = Build Array("Counts", "Absorbance (au)", "% Transmission", "Irradiance (Watts/m^2)") -> (w336:string[])
              n184 = Index Array(array=w336, index=w335) -> (element=w334:string)
              n185 = local read "ChartView"() -> (w331:T3)
              n186 = case "Populates  Reference Array" shown="True" "Take Reference" {
                tunnel: w322 -> [_ w351]
                frame False {
                }
                frame True {
                  n187 = global write "StellarNet SpectraWiz Globals.vi" "[reference]"(w351) -> ()
                }
              }
              n188 = case "Populates  Dark Array" shown="True" "Take Dark" {
                tunnel: w322 -> [_ w350]
                frame False {
                }
                frame True {
                  n189 = global write "StellarNet SpectraWiz Globals.vi" "[dark]"(w350) -> ()
                  n190 = local write "Use Dark"(TRUE ("Use Dark")) -> ()
                }
              }
              n191 = property class="XYGraph (strict)"("Y Scale.Name Label.Text"=w334) -> ()  [unwired: 2 in, 2 out]
              n192 = property class="XYGraph (strict)"("Y Scale.Name Label.Text"=w334) -> ()  [unwired: 2 in, 2 out]
              n193 = call "File Stamp.vi"("ChartView"=w331, "File Stamp"="Create and Log to Time Series Log File", "Time [s]"=w343, "Error In"=w326, "File Path In"=w344) -> ("File Path Out"=w342:path, "Error Out"=w329:errorcluster)  [unwired: 9 in]
            }
          }
          n194 = local read "Stop Program"() -> (w106:bool)
          n195 = Not(x=w106) -> (.not. x?=w105:bool)
          n196 = Unbundle By Name(w117) -> ("status"=w111:bool)
          n197 = Not(x=w111) -> (.not. x?=w110:bool)
          n198 = Compound Arithmetic op=AND(w110, w109, w105) -> (w108:bool)
          n199 = Not(x=w108) -> (.not. x?=w107:bool)
          n200 = global write "StellarNet SpectraWiz Globals.vi" "Global Stop"(w107) -> ()
        }
        n201 = while {
          tunnel: w57 -> [_]
          stop <- w87 stop-if-true
          # "DAEMON LOOP"
          # "Parallel loop implements 1-based \"indexing\" for the \nchannel parameters (so channels are labeled 1...N)\nand provides a global stop button that terminates\nexecution after each state in the state machine."
          n202 = flat-sequence {
            tunnel: [w94] -> w89
            tunnel: ["Stop Program"] -> w88
            frame #0 {
              n203 = global read "StellarNet SpectraWiz Globals.vi" "Global Stop"() -> (w94:bool)
            }
            frame #1 {
              n204 = global write "StellarNet SpectraWiz Globals.vi" "Global Stop"("Stop Program") -> ()
            }
          }
          n205 = local read "Channel"() -> (w92:u8)
          n206 = Decrement(x=w92) -> (x-1=w91:u8)
          n207 = Build Array(w91) -> (w90:u8[])
          n208 = property on="Operating Parameters" class="Arr (strict)"("Index Values"=w90) -> ()  [unwired: 2 in, 2 out]
          n209 = Or(x=w89, y=w88) -> (x .or. y?=w87:bool)
          n210 = Wait (ms)(milliseconds to wait=u32 100) -> ()  [unwired: 1 out]
        }
      }
    }
  }
  n211 = call <vilib>:"Simple Error Handler.vi"("error in (no error)"=w1) -> ()  [unwired: 4 in, 5 out]
